vi "Dodanie położeń robotów do mapy.vi"(0 "Mapa terenu":picture, 1 "Rozmiar mapy":T5={"left"=0, "top"=0, "right"=836, "bottom"=597}, 5 "Wybór robota":T7 items=["Łazik", "Quadron", "Dron 1", "Dron 2"], 7 "Poł. bazowe\n piksele":cluster{"X":i32, "Y":i32}, 11 "Właściwości mapy":T4={"Przesunięcie mapy"={"X"=0, "Y"=0}, "Dł. px[m]"=0.19634281539316645, "Zoom mapy"=1.0, "Wpisane punkty na\nliście współrzędnych"=983260, "Zaznaczony punkt"=16448250, "Układ współrzędnych"=323328, "Początkowe położenie robota"=16448250, "Trasa robota - Łazik"=2815743, "Ost. zazn. pkt"={"X"=0, "Y"=0}, "Draw Area Size"={"Width"=528, "Height"=564}} {"Zoom mapy" scale=0.2..6.0}, 12 "Skalowanie i kolory":T1={"Polozenie 1"={"X"=265, "Y"=265}, "  Wybór \nznacznika"=FALSE, "   Polozenie 2"={"X"=358, "Y"=265}, "   Blokada \nznaczników"=FALSE, "Kolor  znaczników"=16774930, "Grubość \nznaczników"=2, "Wyznaczanie odległości"=enum."Odległość pomiędzy znacznikami", "Współrzędne geograficzne 1"="", "Współrzędne geograficzne 2"="", "Odl. pomiędzy znacznikami [m]"=15.0}, 13 "Lokalizacja robotów":T2, 14 "Legenda":T6={"Łazik"=16318208, "Quadron"=16318208, "Dron 1"=16318208, "Dron 2"=16318208, "Sparus"=16318208}) -> (4 "Mapa terenu stała":picture, 6 "Mapa terenu wyświetlana":picture)   [LabVIEW 2015, in "Biblioteka moduł map v3.lvlib" / "Pomocnicze.lvlib"]
uses:
  Pomocnicze.lvlib
  <vilib>/Utility/miscctls.llb/LVBoundsTypeDef.ctl
  Kontrolki/Kontrolki.lvlib
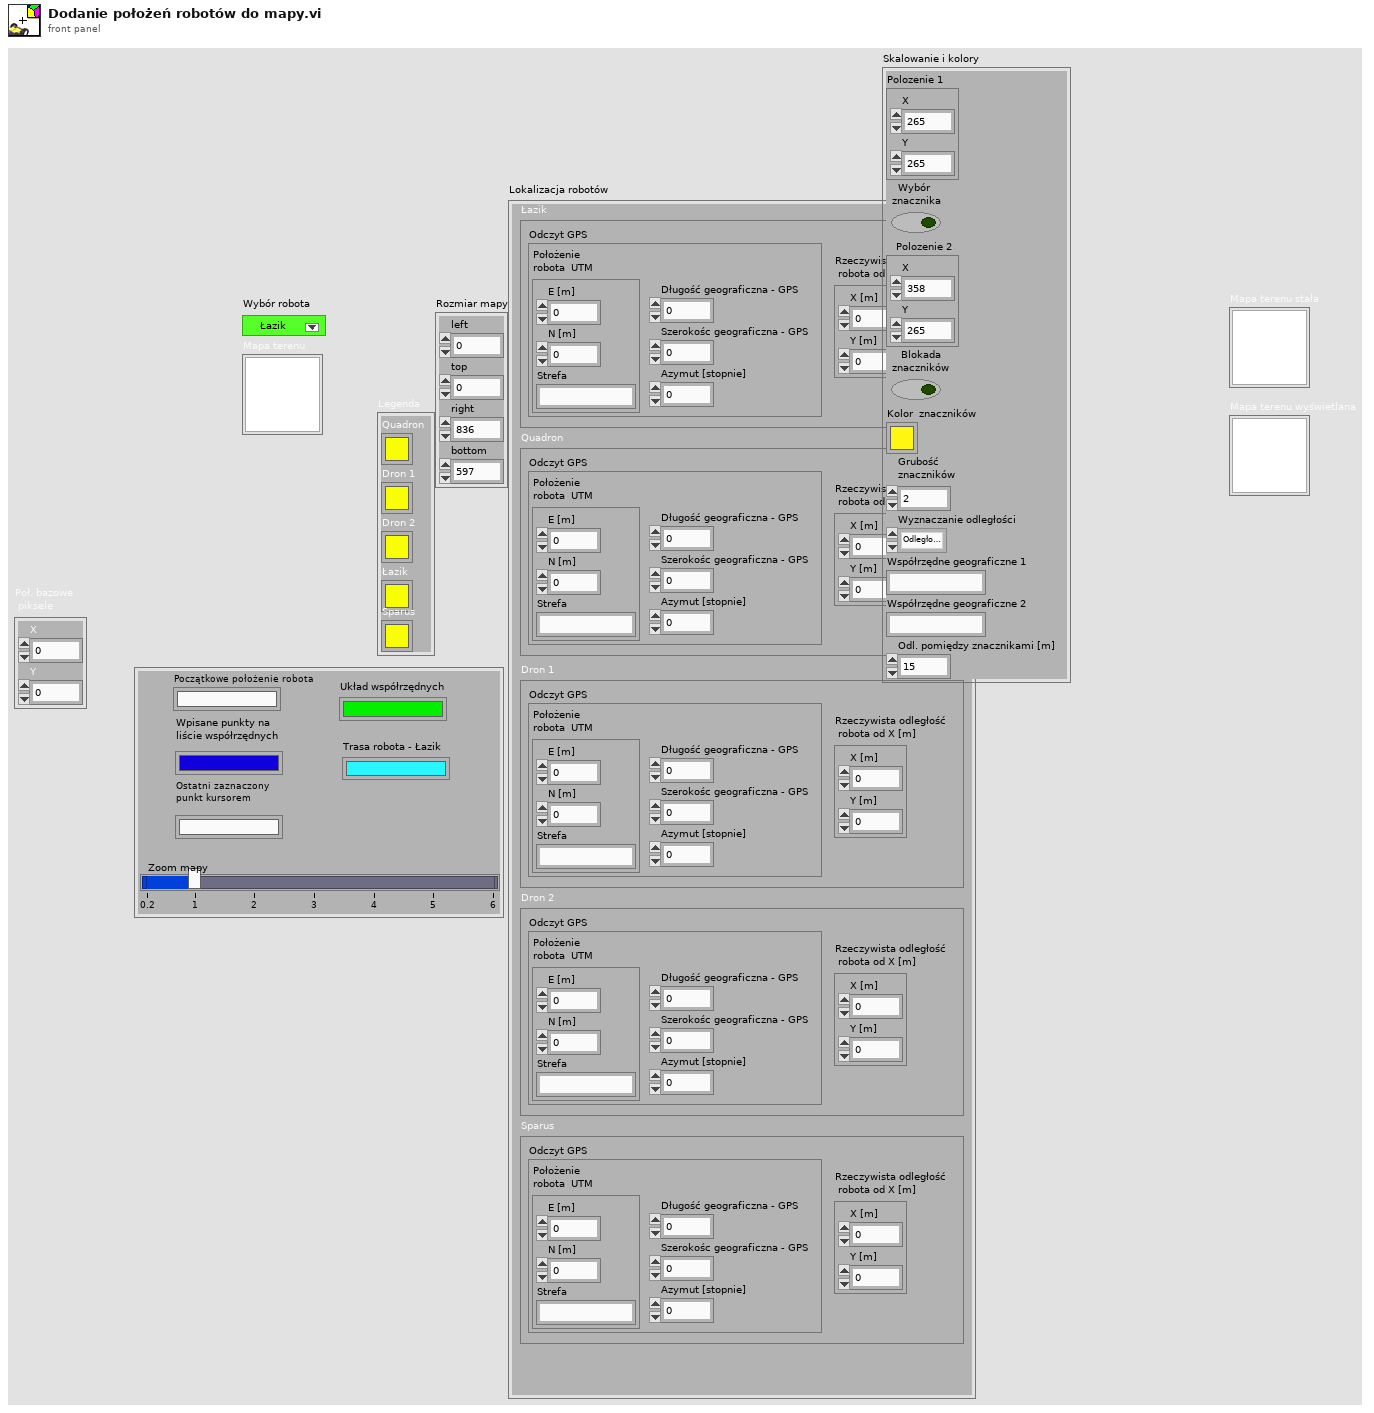
[diagram p1: front panel]
types:
  T1 = cluster{"Polozenie 1":cluster{"X":i32, "Y":i32}, "  Wybór \nznacznika":bool, "   Polozenie 2":cluster{"X":i32, "Y":i32}, "   Blokada \nznaczników":bool, "Kolor  znaczników":u32, "Grubość \nznaczników":u32, "Wyznaczanie odległości":enum16{"Współrzędne geograficzne", "Odległość pomiędzy znacznikami"}, "Współrzędne geograficzne 1":string, "Współrzędne geograficzne 2":string, "Odl. pomiędzy znacznikami [m]":dbl}
  T2 = typedef "Biblioteka moduł map v3.lvlib/Kontrolki.lvlib/Lokalizacja robotów.ctl" = cluster{"Łazik":cluster{"Odczyt GPS":cluster{"Położenie \nrobota  UTM":cluster{"E [m]":ext, "N [m]":ext, "Strefa":string}, "Długość geograficzna - GPS":dbl, "Szerokośc geograficzna - GPS":dbl, "Azymut [stopnie]":dbl}, "Rzeczywista odległość\n robota od X [m]":cluster{"X [m]":dbl, "Y [m]":dbl}}, "Quadron":cluster{"Odczyt GPS":cluster{"Położenie \nrobota  UTM":cluster{"E [m]":ext, "N [m]":ext, "Strefa":string}, "Długość geograficzna - GPS":dbl, "Szerokośc geograficzna - GPS":dbl, "Azymut [stopnie]":dbl}, "Rzeczywista odległość\n robota od X [m]":cluster{"X [m]":dbl, "Y [m]":dbl}}, "Dron 1":cluster{"Odczyt GPS":cluster{"Położenie \nrobota  UTM":cluster{"E [m]":ext, "N [m]":ext, "Strefa":string}, "Długość geograficzna - GPS":dbl, "Szerokośc geograficzna - GPS":dbl, "Azymut [stopnie]":dbl}, "Rzeczywista odległość\n robota od X [m]":cluster{"X [m]":dbl, "Y [m]":dbl}}, "Dron 2":cluster{"Odczyt GPS":cluster{"Położenie \nrobota  UTM":cluster{"E [m]":ext, "N [m]":ext, "Strefa":string}, "Długość geograficzna - GPS":dbl, "Szerokośc geograficzna - GPS":dbl, "Azymut [stopnie]":dbl}, "Rzeczywista odległość\n robota od X [m]":cluster{"X [m]":dbl, "Y [m]":dbl}}, "Sparus":cluster{"Odczyt GPS":cluster{"Położenie \nrobota  UTM":cluster{"E [m]":ext, "N [m]":ext, "Strefa":string}, "Długość geograficzna - GPS":dbl, "Szerokośc geograficzna - GPS":dbl, "Azymut [stopnie]":dbl}, "Rzeczywista odległość\n robota od X [m]":cluster{"X [m]":dbl, "Y [m]":dbl}}}
  T3 = typedef "LVBoundsTypeDef.ctl" = cluster{"Width":u32, "Height":u32}
  T4 = cluster{"Przesunięcie mapy":cluster{"X":i16, "Y":i16}, "Dł. px[m]":dbl, "Zoom mapy":sgl, "Wpisane punkty na\nliście współrzędnych":u32, "Zaznaczony punkt":u32, "Układ współrzędnych":u32, "Początkowe położenie robota":u32, "Trasa robota - Łazik":u32, "Ost. zazn. pkt":cluster{"X":i32, "Y":i32}, "Draw Area Size":T3}
  T5 = cluster{"left":i16, "top":i16, "right":i16, "bottom":i16}
  T6 = cluster{"Łazik":u32, "Quadron":u32, "Dron 1":u32, "Dron 2":u32, "Sparus":u32}
  T7 = typedef "Biblioteka moduł map v3.lvlib/Kontrolki.lvlib/Wybór robota.ctl" = u16
  T8 = cluster{"Rozmiar mapy":cluster{"Szerokość":i16, "Wysokość":i16}, "Dł. piksela [m]":dbl, "Trasa robota":u32, "Poł. bazowe\n piksele":cluster{"X":i32, "Y":i32}}
  T9 = cluster{"Odl. robota od startu [m]":cluster{"X":dbl, "Y":dbl}, "Położenie startowe":cluster{"X":i32, "Y":i32}, "Azymut [stopnie]":dbl}
  T10 = cluster{"Położenie  środka":cluster{"Pixel x":i16, "Pixel y":i16}, "Kolor ":u32, "Grubość  ":u32}
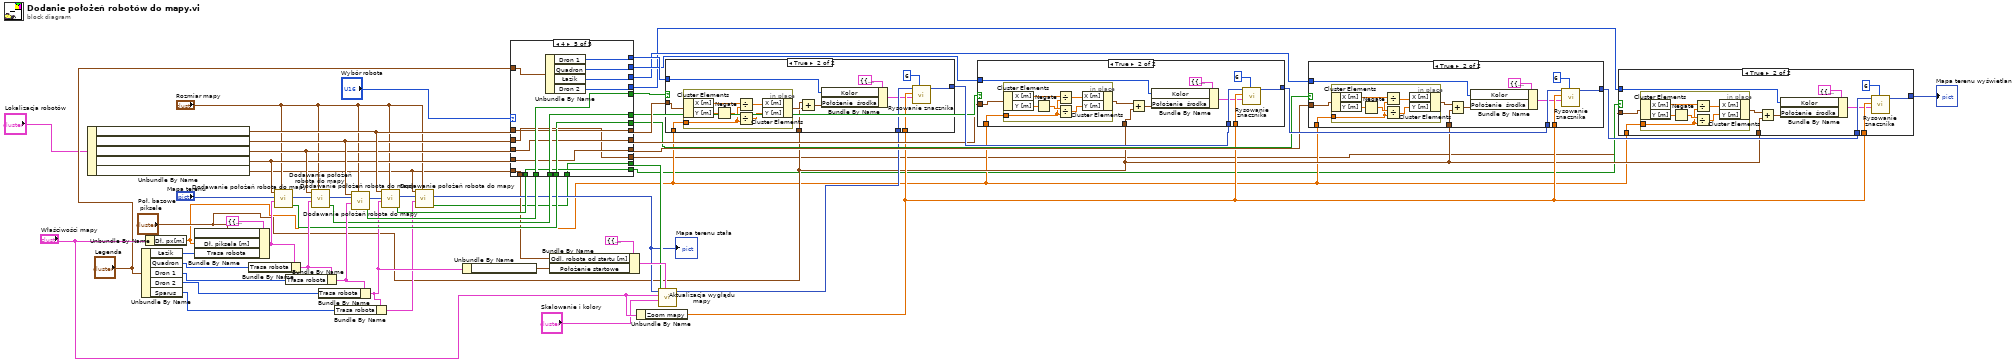
[diagram p0: block diagram]
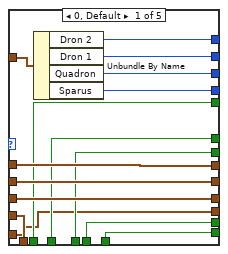
[diagram p6: hidden frame]
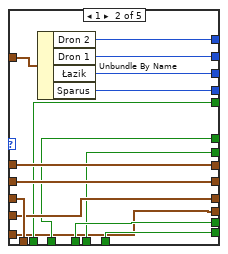
[diagram p7: hidden frame]
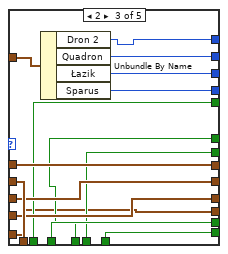
[diagram p8: hidden frame]
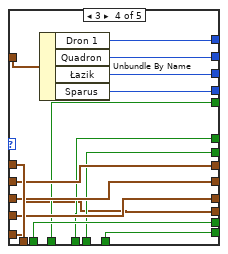
[diagram p9: hidden frame]
diagram:
  n1 = Unbundle By Name("Lokalizacja robotów") -> ("Dron 2.Rzeczywista odległość\n robota od X [m]"=w35:cluster{"X [m]":dbl, "Y [m]":dbl}, "Dron 1.Rzeczywista odległość\n robota od X [m]"=w34:cluster{"X [m]":dbl, "Y [m]":dbl}, "Quadron.Rzeczywista odległość\n robota od X [m]"=w33:cluster{"X [m]":dbl, "Y [m]":dbl}, "Łazik.Rzeczywista odległość\n robota od X [m]"=w32:cluster{"X [m]":dbl, "Y [m]":dbl}, "Sparus.Rzeczywista odległość\n robota od X [m]"=w10:cluster{"X [m]":dbl, "Y [m]":dbl})
  n2 = Unbundle By Name("Legenda") -> ("Łazik"=w53:u32, "Quadron"=w49:u32, "Dron 1"=w48:u32, "Dron 2"=w47:u32, "Sparus"=w15:u32)
  n3 = Unbundle By Name("Właściwości mapy") -> ("Dł. px[m]"=w5:dbl)
  n4 = Bundle By Name(cluster=T8 {"Rozmiar mapy"={"Szerokość"=0, "Wysokość"=0}, "Dł. piksela [m]"=0.19634281539316645, "Trasa robota"=16722479, "Poł. bazowe\n piksele"={"X"=0, "Y"=0}} ("Dane do wyzn. poł. robota na mapie 2"), "Poł. bazowe\n piksele"="Poł. bazowe\n piksele", "Dł. piksela [m]"=w5, "Trasa robota"=w53) -> (w52:T8)
  n5 = Bundle By Name(cluster=w52, "Trasa robota"=w49) -> (w51:T8)
  n6 = call "Dodawanie położeń robota do mapy.vi"("Rozmiar mapy"="Rozmiar mapy", "Dane do wyzn. poł. robota na mapie"=w52, "Mapa terenu"="Mapa terenu", "Odl. robota od startu"=w32) -> ("Pol. w zakresie mapy"=w39:bool, "Mapa z wprowadzonym punktem"=w57:picture)  [unwired: 5 in, 1 out]
  n7 = Bundle By Name(cluster=w51, "Trasa robota"=w48) -> (w50:T8)
  n8 = call "Dodawanie położeń robota do mapy.vi"("Rozmiar mapy"="Rozmiar mapy", "Dane do wyzn. poł. robota na mapie"=w51, "Mapa terenu"=w57, "Odl. robota od startu"=w33) -> ("Pol. w zakresie mapy"=w38:bool, "Mapa z wprowadzonym punktem"=w56:picture)  [unwired: 5 in, 1 out]
  n9 = Bundle By Name(cluster=w50, "Trasa robota"=w47) -> (w16:T8)
  n10 = Bundle By Name(cluster=w16, "Trasa robota"=w15) -> (w14:T8)
  n11 = call "Dodawanie położeń robota do mapy.vi"("Rozmiar mapy"="Rozmiar mapy", "Dane do wyzn. poł. robota na mapie"=w50, "Mapa terenu"=w56, "Odl. robota od startu"=w34) -> ("Pol. w zakresie mapy"=w37:bool, "Mapa z wprowadzonym punktem"=w55:picture)  [unwired: 5 in, 1 out]
  n12 = call "Dodawanie położeń robota do mapy.vi"("Rozmiar mapy"="Rozmiar mapy", "Dane do wyzn. poł. robota na mapie"=w16, "Mapa terenu"=w55, "Odl. robota od startu"=w35) -> ("Pol. w zakresie mapy"=w36:bool, "Mapa z wprowadzonym punktem"=w18:picture)  [unwired: 5 in, 1 out]
  n13 = call "Dodawanie położeń robota do mapy.vi"("Rozmiar mapy"="Rozmiar mapy", "Dane do wyzn. poł. robota na mapie"=w14, "Mapa terenu"=w18, "Odl. robota od startu"=w10) -> ("Pol. w zakresie mapy"=w11:bool, "Mapa z wprowadzonym punktem"=w17:picture)  [unwired: 5 in, 1 out]
  "Mapa terenu stała" <- w17
  n14 = Unbundle By Name(w16) -> ("Poł. bazowe\n piksele"=w45:cluster{"X":i32, "Y":i32})
  n15 = case shown="4" "Wybór robota" {
    tunnel: w32 -> [w73 w85 w99 w111 w121]
    tunnel: w33 -> [w70 w88 w100 w112 w122]
    tunnel: w34 -> [w71 w86 w103 w113 w123]
    tunnel: w35 -> [w72 w87 w101 w118 w119]
    tunnel: [w73 w88 w103 w118 w133] -> w12
    tunnel: [w72 w87 w101 w113 w123] -> w30
    tunnel: [w71 w86 w100 w112 w122] -> w23
    tunnel: [w70 w85 w99 w111 w121] -> w22
    tunnel: "Legenda" -> [w69 w84 w102 w117 w132]
    tunnel: [w68 w81 w96 w114 w129] -> w25
    tunnel: [w67 w82 w97 w115 w130] -> w26
    tunnel: [w66 w83 w98 w116 w131] -> w29
    tunnel: [w65 w80 w95 w110 w120] -> w40
    tunnel: w39 -> [w65 w77 w92 w107 w125]
    tunnel: w38 -> [w62 w80 w93 w108 w126]
    tunnel: w37 -> [w63 w78 w95 w109 w127]
    tunnel: w36 -> [w64 w79 w94 w110 w124]
    tunnel: [w64 w79 w94 w109 w127] -> w31
    tunnel: [w63 w78 w93 w108 w126] -> w24
    tunnel: [w62 w77 w92 w107 w125] -> w21
    tunnel: w11 -> [w60 w75 w90 w105 w120]
    tunnel: w10 -> [w59 w74 w89 w104 w133]
    tunnel: [w61 w76 w91 w106 w128] -> w4
    tunnel: [w60 w75 w90 w105 w124] -> w3
    tunnel: [w59 w74 w89 w104 w119] -> w2
    frame 0, Default {
      n16 = Unbundle By Name(w69) -> ("Dron 2"=w66:u32, "Dron 1"=w67:u32, "Quadron"=w68:u32, "Sparus"=w61:u32)
    }
    frame 1 {
      n17 = Unbundle By Name(w84) -> ("Dron 2"=w83:u32, "Dron 1"=w82:u32, "Łazik"=w81:u32, "Sparus"=w76:u32)
    }
    frame 2 {
      n18 = Unbundle By Name(w102) -> ("Dron 2"=w98:u32, "Quadron"=w97:u32, "Łazik"=w96:u32, "Sparus"=w91:u32)
    }
    frame 3 {
      n19 = Unbundle By Name(w117) -> ("Dron 1"=w116:u32, "Quadron"=w115:u32, "Łazik"=w114:u32, "Sparus"=w106:u32)
    }
    frame 4 {
      n20 = Unbundle By Name(w132) -> ("Dron 1"=w131:u32, "Quadron"=w130:u32, "Łazik"=w129:u32, "Dron 2"=w128:u32)
    }
  }
  n21 = Bundle By Name(cluster=T9 {"Odl. robota od startu [m]"={"X"=246.0, "Y"=243.0}, "Położenie startowe"={"X"=246, "Y"=243}, "Azymut [stopnie]"=297.94899101038743} ("Położenie robota"), "Odl. robota od startu [m]"=w12, "Położenie startowe"=w45) -> (w44:T9)
  n22 = Unbundle By Name("Właściwości mapy") -> ("Zoom mapy"=w8:sgl)
  n23 = call "Aktualizacja wyglądu mapy.vi"("Położenie robota"=w44, "Poł. w zakresie mapy"=w40, "Skalowanie i kolory"="Skalowanie i kolory", "Właściwości mapy"="Właściwości mapy", "Mapa"=w17) -> ("Przesunięta mapa"=w20:picture)  [unwired: 6 in]
  n24 = case shown="True" w31 {
    tunnel: w20 -> [w134 w145]
    tunnel: w8 -> [_ w144]
    tunnel: w30 -> [_ w138]
    tunnel: w29 -> [_ w141]
    tunnel: w5 -> [_ w137]
    tunnel: "Poł. bazowe\n piksele" -> [_ w135]
    tunnel: [w134 w139] -> w27
    frame False {
    }
    frame True {
      n25 = in-place {
        in-place-border: w137 -> [w147]
        n26 = in-place-cluster #1(w138) -> ("X [m]"=w152:dbl, "Y [m]"=w148:dbl)
        n27 = Negate(x=w148) -> (-x=w149:dbl)
        n28 = Divide(x=w152, y=w147) -> (x/y=w151:dbl)
        n29 = Divide(x=w149, y=w147) -> (x/y=w150:dbl)
        n30 = in-place-cluster #1("X [m]"=w151, "Y [m]"=w150) -> (w136:cluster{"X [m]":dbl, "Y [m]":dbl})
      }
      n31 = Add(x=w136, y=w135) -> (x+y=w142:cluster{dbl, dbl})
      n32 = Bundle By Name(cluster=T10 {"Położenie  środka"={"Pixel x"=0, "Pixel y"=0}, "Kolor "=0, "Grubość  "=2} ("Znacznik na mapie"), "Kolor"=w141, "Położenie  środka"=w142) -> (w140:T10)
      n33 = call "Rysowanie znacznika.vi"("Rozmiar znacznika"=6, "Znacznik na mapie"=w140, "Zoom mapy"=w144, "Mapa terenu"=w145) -> ("Mapa z wprowadzonym znacznikiem"=w139:picture)  [unwired: 7 in]
    }
  }
  n34 = case shown="True" w24 {
    tunnel: w27 -> [w153 w164]
    tunnel: w8 -> [_ w163]
    tunnel: w23 -> [_ w156]
    tunnel: w26 -> [_ w160]
    tunnel: w5 -> [_ w155]
    tunnel: [w153 w158] -> w28
    tunnel: "Poł. bazowe\n piksele" -> [_ w157]
    frame False {
    }
    frame True {
      n35 = in-place {
        in-place-border: w155 -> [w166]
        n36 = in-place-cluster #2(w156) -> ("X [m]"=w171:dbl, "Y [m]"=w167:dbl)
        n37 = Negate(x=w167) -> (-x=w168:dbl)
        n38 = Divide(x=w171, y=w166) -> (x/y=w170:dbl)
        n39 = Divide(x=w168, y=w166) -> (x/y=w169:dbl)
        n40 = in-place-cluster #2("X [m]"=w170, "Y [m]"=w169) -> (w154:cluster{"X [m]":dbl, "Y [m]":dbl})
      }
      n41 = Add(x=w154, y=w157) -> (x+y=w161:cluster{dbl, dbl})
      n42 = Bundle By Name(cluster=T10 {"Położenie  środka"={"Pixel x"=0, "Pixel y"=0}, "Kolor "=0, "Grubość  "=2} ("Znacznik na mapie"), "Kolor"=w160, "Położenie  środka"=w161) -> (w159:T10)
      n43 = call "Rysowanie znacznika.vi"("Rozmiar znacznika"=6, "Znacznik na mapie"=w159, "Zoom mapy"=w163, "Mapa terenu"=w164) -> ("Mapa z wprowadzonym znacznikiem"=w158:picture)  [unwired: 7 in]
    }
  }
  n44 = case shown="True" w21 {
    tunnel: w28 -> [w172 w183]
    tunnel: w8 -> [_ w182]
    tunnel: w22 -> [_ w174]
    tunnel: w25 -> [_ w179]
    tunnel: w5 -> [_ w173]
    tunnel: "Poł. bazowe\n piksele" -> [_ w178]
    tunnel: [w172 w176] -> w7
    frame False {
    }
    frame True {
      n45 = in-place {
        in-place-border: w173 -> [w185]
        n46 = in-place-cluster #3(w174) -> ("X [m]"=w190:dbl, "Y [m]"=w186:dbl)
        n47 = Negate(x=w186) -> (-x=w187:dbl)
        n48 = Divide(x=w190, y=w185) -> (x/y=w189:dbl)
        n49 = Divide(x=w187, y=w185) -> (x/y=w188:dbl)
        n50 = in-place-cluster #3("X [m]"=w189, "Y [m]"=w188) -> (w175:cluster{"X [m]":dbl, "Y [m]":dbl})
      }
      n51 = Add(x=w175, y=w178) -> (x+y=w180:cluster{dbl, dbl})
      n52 = Bundle By Name(cluster=T10 {"Położenie  środka"={"Pixel x"=0, "Pixel y"=0}, "Kolor "=0, "Grubość  "=2} ("Znacznik na mapie"), "Kolor"=w179, "Położenie  środka"=w180) -> (w177:T10)
      n53 = call "Rysowanie znacznika.vi"("Rozmiar znacznika"=6, "Znacznik na mapie"=w177, "Zoom mapy"=w182, "Mapa terenu"=w183) -> ("Mapa z wprowadzonym znacznikiem"=w176:picture)  [unwired: 7 in]
    }
  }
  n54 = case shown="True" w3 {
    tunnel: w7 -> [w191 w202]
    tunnel: w8 -> [_ w201]
    tunnel: w2 -> [_ w193]
    tunnel: w4 -> [_ w198]
    tunnel: w5 -> [_ w192]
    tunnel: "Poł. bazowe\n piksele" -> [_ w197]
    tunnel: [w191 w195] -> w9
    frame False {
    }
    frame True {
      n55 = in-place {
        in-place-border: w192 -> [w204]
        n56 = in-place-cluster #4(w193) -> ("X [m]"=w209:dbl, "Y [m]"=w205:dbl)
        n57 = Negate(x=w205) -> (-x=w206:dbl)
        n58 = Divide(x=w209, y=w204) -> (x/y=w208:dbl)
        n59 = Divide(x=w206, y=w204) -> (x/y=w207:dbl)
        n60 = in-place-cluster #4("X [m]"=w208, "Y [m]"=w207) -> (w194:cluster{"X [m]":dbl, "Y [m]":dbl})
      }
      n61 = Add(x=w194, y=w197) -> (x+y=w199:cluster{dbl, dbl})
      n62 = Bundle By Name(cluster=T10 {"Położenie  środka"={"Pixel x"=0, "Pixel y"=0}, "Kolor "=0, "Grubość  "=2} ("Znacznik na mapie"), "Kolor"=w198, "Położenie  środka"=w199) -> (w196:T10)
      n63 = call "Rysowanie znacznika.vi"("Rozmiar znacznika"=6, "Znacznik na mapie"=w196, "Zoom mapy"=w201, "Mapa terenu"=w202) -> ("Mapa z wprowadzonym znacznikiem"=w195:picture)  [unwired: 7 in]
    }
  }
  "Mapa terenu wyświetlana" <- w9
